vi "FIFO Manager - Transfer.vi"(7 "timeout in ms (-1)":i32, 9 "Word In":u32, 11 "error in (no error)":errorcluster, 13 "Operation":T1) -> (4 "Data Out":u32, 8 "Timed Out":bool, 15 "error out":errorcluster)   [LabVIEW 2017, in "FPGA-SRL.lvlib"]
uses:
  FPGA-SRL.lvlib
  Type Defs/WSVCAP SHL FIFO Operation Enum.ctl
  <vilib>/rvi/DataTransferAndStorage/Container/XNode/niFpgaContainer.xnode
  <vilib>/rvi/FIFO/Fifo_Resource/nirvififoEmulationRead.vi
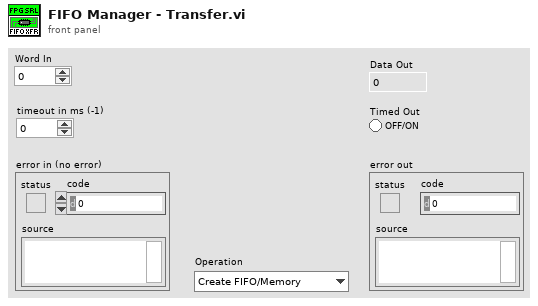
[diagram p1: front panel]
types:
  T1 = typedef "WSVCAP SHL FIFO Operation Enum.ctl" = enum16{"Create FIFO/Memory", "Get Write FIFO Status", "Get Read FIFO Status", "Put Element in Write", "Put Element in Read", "Get Element from Write", "Get Element from Read"}
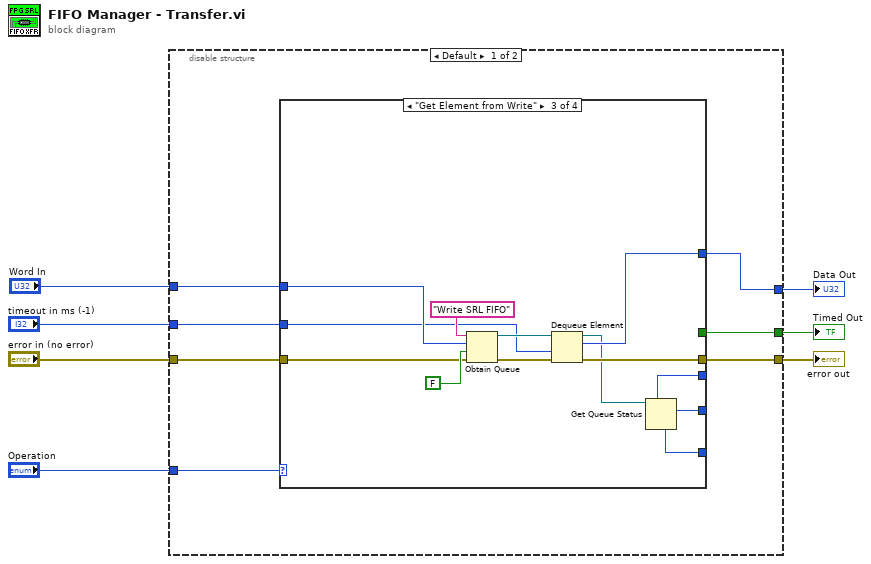
[diagram p0: block diagram]
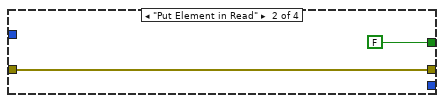
[diagram p3: hidden frame]
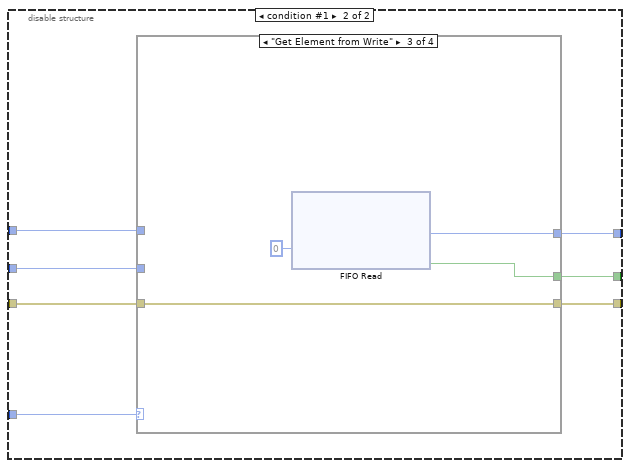
[diagram p5: hidden frame]
diagram:
  n1 = disable-structure shown="Default" {
    disable-tunnel: "Operation" -> [w14 w38]
    disable-tunnel: "error in (no error)" -> [w13 w35]
    disable-tunnel: [w12 w34] -> w5
    disable-tunnel: "timeout in ms (-1)" -> [w11 w37]
    disable-tunnel: [w10 w33] -> w1
    disable-tunnel: [w9 w36] -> w3
    disable-tunnel: "Word In" -> [w8 w32]
    frame condition #0 (active) {
      n2 = case shown="\"Get Element from Write\"" w14 {
        tunnel: [w15 w17 w25 w31] -> w12
        tunnel: w13 -> [w15 w17 w26 w31]
        tunnel: w11 -> [_ _ w23 _]
        tunnel: [_ _ w22 _] -> w10
        tunnel: [_ FALSE _ _] -> w9
        tunnel: w8 -> [_ _ w24 _]
        tunnel: [_ _ w20 _] -> _
        tunnel: [_ _ w19 _] -> _
        tunnel: [_ _ w18 _] -> _
        frame Default {
        }
        frame "Put Element in Read" {
        }
        frame "Get Element from Write" {
          n3 = Obtain Queue(name (unnamed)="Write SRL FIFO", element data type=w24, create if not found? (T)=FALSE, error in (no error)=w26) -> (queue out=w28:refnum<queue>, error out=w30:errorcluster)  [unwired: 1 in, 1 out]
          n4 = Dequeue Element(queue=w28, timeout in ms (-1)=w23, error in (no error)=w30) -> (queue out=w21:refnum<queue>, element=w22:u32, error out=w25:errorcluster)  [unwired: 1 out]
          n5 = Get Queue Status(queue=w21) -> (max queue size=w18:i32, # pending remove=w19:i32, # elements in queue=w20:i32)  [unwired: 2 in, 5 out]
        }
        frame "Get Read FIFO Status" {
        }
      }
    }
    frame condition #1 {
      n6 = case shown="\"Get Element from Write\"" w38 {
        tunnel: w37 -> [_ _ _ _]
        tunnel: [_ _ w41 _] -> w36
        tunnel: w35 -> [w39 w40 w44 w45]
        tunnel: [w39 w40 w44 w45] -> w34
        tunnel: [_ _ w43 _] -> w33
        tunnel: w32 -> [_ _ _ _]
        frame "Put Element in Read" {
        }
        frame Default {
        }
        frame "Get Element from Write" {
          n7 = xnode "FIFO Read"("Timeout"=0) -> ("Element"=w43:u32, "Timed Out?"=w41:bool)  [unwired: 1 in, 1 out]
        }
        frame "Get Read FIFO Status" {
        }
      }
    }
  }
  "error out" <- w5
  "Timed Out" <- w3
  "Data Out" <- w1
